vi "chartxy.vi"(0 "选择调整的轴":enum16{"Y", "X", "X、Y"}(ring), 1 "X标尺.长度":dbl, 2 "Y标尺.最大值":dbl, 3 "曲线数量":u8, 4 "波形图表引用输入":refnum<vi>) -> ()   [LabVIEW 2018]
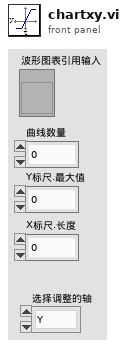
[diagram p1: front panel]
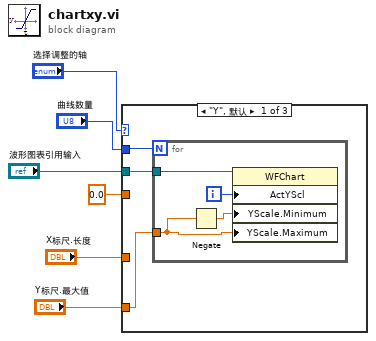
[diagram p0: block diagram]
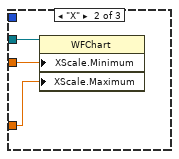
[diagram p2: hidden frame]
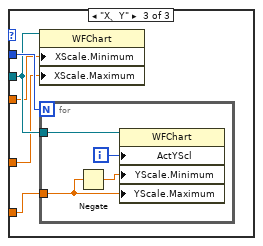
[diagram p3: hidden frame]
diagram:
  n1 = case shown="\"Y\", 默认" "选择调整的轴" {
    tunnel: "曲线数量" -> [w7 _ w21]
    tunnel: "Y标尺.最大值" -> [w8 _ w20]
    tunnel: "波形图表引用输入" -> [w9 w16 w19]
    tunnel: 0.0 ("X标尺.范围:最小值") -> [_ w15 w18]
    tunnel: "X标尺.长度" -> [_ w14 w17]
    frame "Y", Default {
      n2 = for {
        N: w7 -> [_]
        tunnel: w8 -> [w11]
        tunnel: w9 -> [w10]
        i -> [w12]
        n3 = Negate(x=w11) -> (-x=w13:dbl)
        n4 = property on="属性节点" class="WFChart"(reference=w10, "ActYScl"=w12, "YScale.Minimum"=w13, "YScale.Maximum"=w11) -> ()  [unwired: 1 in, 2 out]
      }
    }
    frame "X" {
      n5 = property on="属性节点" class="WFChart"(reference=w16, "XScale.Minimum"=w15, "XScale.Maximum"=w14) -> ()  [unwired: 1 in, 2 out]
    }
    frame "X、Y" {
      n6 = property on="属性节点" class="WFChart"(reference=w19, "XScale.Minimum"=w18, "XScale.Maximum"=w17) -> ()  [unwired: 1 in, 2 out]
      n7 = for {
        N: w21 -> [_]
        tunnel: w20 -> [w23]
        tunnel: w19 -> [w22]
        i -> [w24]
        n8 = Negate(x=w23) -> (-x=w25:dbl)
        n9 = property on="属性节点" class="WFChart"(reference=w22, "ActYScl"=w24, "YScale.Minimum"=w25, "YScale.Maximum"=w23) -> ()  [unwired: 1 in, 2 out]
      }
    }
  }
